vi "ProdaNG.TestSteps.Get.vi"(8 "error in (no error)":errorcluster, 9 "orderby (Test Sequence)":T1, 10 "processStepId":i32, 11 "dbHandleIn":i32) -> (0 "error out":errorcluster, 2 "TestSteps":T2[](array[typedef]), 3 "dbHandle":i32)   [LabVIEW 2016]
doc: "This function returns a product structure for a product, which is identified by a part and a serial number.\nImportant information: The field 'individual' was taken over from the field 'allgemein' of the legacy data directly. Because of this most products have the value 0 further on and only a few the value 1. \nParameter:\nhandle is an Integer, which is returned by the function Login() at the creation of a new connection.\nwabcoPartId is the Id of the part.\nserialNumber is the serial number of the product for the part above.\nproduct is a pointer on a product structure, which is filled if the returncode is 0. The structure must be defined in the calling program.\n\nReturncodes:\n0 No error\n< 0 ORACLE Error code\n6 (ERROR_INVALID_HANDLE) in case of an invalid handle\n1403 Record does not exist"
uses:
  Controls/ProdaNG.TestStep.ctl
  Controls/ProdaNG.TestStepOrder.ctl
  Controls/ProdaNG.TestStepSize.ctl
  <vilib>/Utility/importsl/GetValueByPointer/datatype.ctl
  <vilib>/Utility/importsl/GetValueByPointer/GetValueByPointer.xnode
  prodllNG.dll
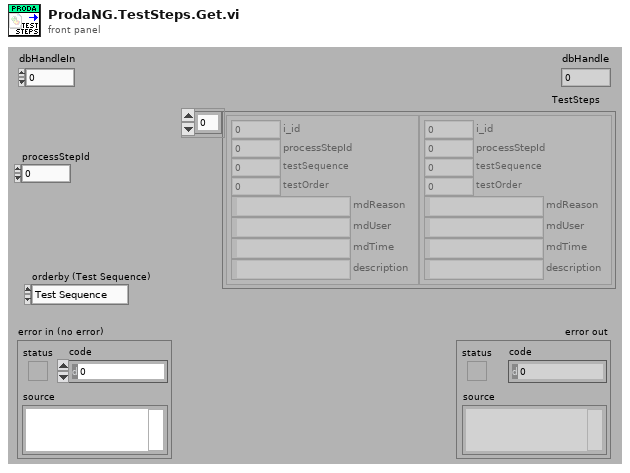
[diagram p1: front panel]
types:
  T1 = typedef "ProdaNG.TestStepOrder.ctl" = enum8{"Test Sequence", "Test Order"}
  T2 = typedef "ProdaNG.TestStep.ctl" = cluster{"i_id":i32, "processStepId":i32, "testSequence":i32, "testOrder":i32, "mdReason":string, "mdUser":string, "mdTime":string, "description":string}
  T3 = typedef "ProdaNG.TestStepSize.ctl" = cluster{"i_id":i32, "processStepId":i32, "testSequence":i32, "testOrder":i32, "mdReason":i32, "mdUser":i32, "mdTime":i32, "description":i32}
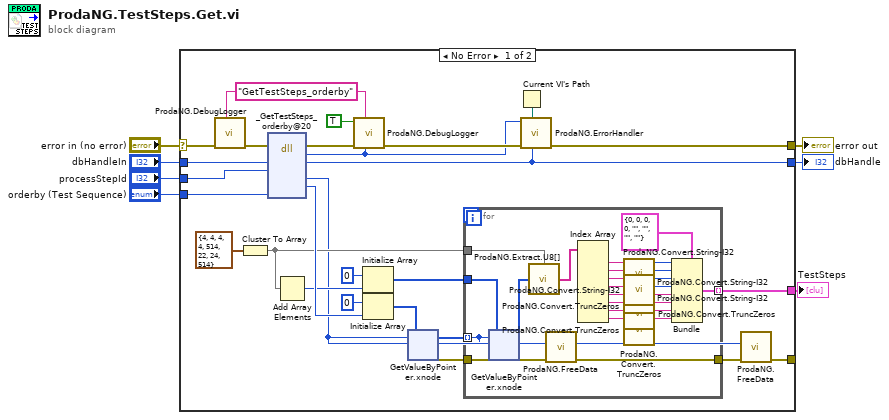
[diagram p0: block diagram]
diagram:
  n1 = case shown="No Error" "error in (no error)" {
    selector: "error in (no error)" -> [w29 w92]
    tunnel: [w34 w92] -> w6
    tunnel: "dbHandleIn" -> [w31 w91]
    tunnel: [w32 w91] -> w4
    tunnel: "processStepId" -> [w16 _]
    tunnel: [w12 _] -> w2
    tunnel: [w9 _] -> _
    tunnel: "orderby (Test Sequence)" -> [w8 _]
    frame No Error {
      w25 = "GetTestSteps_orderby" ("cmd")
      n2 = call "ProdaNG.DebugLogger.vi"("cmd"=w25, "error in (no error)"=w29) -> ("error out"=w28:errorcluster)  [unwired: 9 in]
      n3 = Cluster To Array(cluster=T3 {"i_id"=4, "processStepId"=4, "testSequence"=4, "testOrder"=4, "mdReason"=514, "mdUser"=22, "mdTime"=24, "description"=514} ("TestStepSize")) -> (array=w13:i32[])
      n4 = dll-call lib="D:/Maszup/WABCO/SVN/LineTraceSystem/SOFTWARE/sources/Database/ProdaNG/prodllNG.dll" fn="_GetTestSteps_orderby@20" ("ProDLL wrapper.dll:ProDLL_wrapper_GetWabcoParts_GetData")(error in=w28, "dbHandle"=w31, "processStepId"=w16, "orderby"=w8) -> (error out=w27:errorcluster, "return type"=w24:i32, "dbHandle"=w32:i32, "testStepsPtr"=w10:u32, "countPtr"=w19:i32)  [unwired: 6 in, 1 out]
      n5 = Add Array Elements(numeric array=w13) -> (sum=w15:i32)
      n6 = call "ProdaNG.DebugLogger.vi"("return type"=w24, "cmd"=w25, "error in (no error)"=w27, "done? (F)"=TRUE) -> ("error out"=w26:errorcluster)  [unwired: 7 in]
      n7 = Initialize Array(u8 0 ("element"), w15) -> (w17:u8[])
      n8 = Initialize Array(u32 0 ("element"), w19) -> (w23:u32[])
      n9 = xnode "GetValueByPointer.xnode"("Pointer"=w10, "InputType"=w23) -> ("Output"=w20:u32[], "ErrorOut"=w21:errorcluster)  [unwired: 2 in]
      n10 = for {
        tunnel: w21 -> [w60]
        tunnel: w20 -> [w37] mode=indexing
        tunnel: w17 -> [w59]
        tunnel: w13 -> [w43]
        tunnel: [w42] -> w12 mode=indexing
        tunnel: [w35] -> w11
        n11 = xnode "GetValueByPointer.xnode"("Pointer"=w37, "InputType"=w59, "ErrorIn"=w60) -> ("Output"=w45:u8[], "ErrorOut"=w36:errorcluster)  [unwired: 1 in]
        n12 = call "ProdaNG.Extract.U8[].vi"("unsigned byte array"=w45, "Sizes"=w43) -> ("Elements"=w44:string[])
        n13 = call "ProdaNG.FreeData.vi"("error in (no error)"=w36, "Pointers"=w37) -> ("error out"=w35:errorcluster)  [unwired: 9 in]
        n14 = Index Array(array=w44) -> (element #1=w47:string, element #2=w46:string, element #3=w57:string, element #4=w54:string, element #5=w51:string, element #6=w53:string, element #7=w41:string, element #8=w40:string)  [unwired: 8 in]
        n15 = call "ProdaNG.Convert.String-I32.vi"("unsigned byte string"=w47) -> ("32bit integer"=w49:i32)  [unwired: 10 in]
        n16 = call "ProdaNG.Convert.String-I32.vi"("unsigned byte string"=w46) -> ("32bit integer"=w48:i32)  [unwired: 10 in]
        n17 = call "ProdaNG.Convert.String-I32.vi"("unsigned byte string"=w57) -> ("32bit integer"=w56:i32)  [unwired: 10 in]
        n18 = call "ProdaNG.Convert.String-I32.vi"("unsigned byte string"=w54) -> ("32bit integer"=w55:i32)  [unwired: 10 in]
        n19 = call "ProdaNG.Convert.TruncZeros.vi"("string with \\0s"=w51) -> ("LV string"=w50:string)  [unwired: 10 in]
        n20 = call "ProdaNG.Convert.TruncZeros.vi"("string with \\0s"=w53) -> ("LV string"=w52:string)  [unwired: 10 in]
        n21 = call "ProdaNG.Convert.TruncZeros.vi"("string with \\0s"=w41) -> ("LV string"=w39:string)  [unwired: 10 in]
        n22 = call "ProdaNG.Convert.TruncZeros.vi"("string with \\0s"=w40) -> ("LV string"=w38:string)  [unwired: 10 in]
        n23 = Bundle(cluster=T2 {"i_id"=0, "processStepId"=0, "testSequence"=0, "testOrder"=0, "mdReason"="", "mdUser"="", "mdTime"="", "description"=""} ("TestStep"), "i_id"=w49, "processStepId"=w48, "testSequence"=w56, "testOrder"=w55, "mdReason"=w50, "mdUser"=w52, "mdTime"=w39, "description"=w38) -> (w42:T2)
      }
      n24 = Current VI's Path() -> (path=w33:path)
      n25 = call "ProdaNG.ErrorHandler.vi"("dbHandleIn"=w32, "Path"=w33, "error in"=w26, "output_parameter"=w24) -> ("error out"=w34:errorcluster)  [unwired: 7 in]
      n26 = call "ProdaNG.FreeData.vi"("error in (no error)"=w11, "Pointers"=w10) -> ("error out"=w9:errorcluster)  [unwired: 9 in]
    }
    frame Error {
    }
  }
  "error out" <- w6
  "dbHandle" <- w4
  "TestSteps" <- w2
